vi "Write to Filter Log.vi"(8 "error in (no error)":errorcluster, 11 "Message Log in":refnum<class "Message Log.lvclass">) -> (0 "error out":errorcluster, 3 "Message Log out":refnum<class "Message Log.lvclass">)   [LabVIEW 2017, in "Message Log.lvclass"]
uses:
  Message Log.lvclass
  Message Log.lvclass/Message Log.ctl
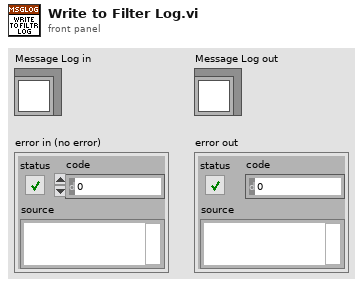
[diagram p1: front panel]
types:
  T1 = typedef "Message Log.lvclass/Message Log Filter Data.ctl" = cluster{"Element":string, "Column":T2, "Filter Type":T3}
  T2 = typedef "Message Log.lvclass/Message Log Columns.ctl" = enum16{"Count (sec)", "Time/Date", "Enque Worker", "Enque Case", "Deque Worker", "Deque Case", "Priority", "Message"}
  T3 = typedef "Message Log.lvclass/String Filter Type.ctl" = enum16{"string only", "match pattern"}
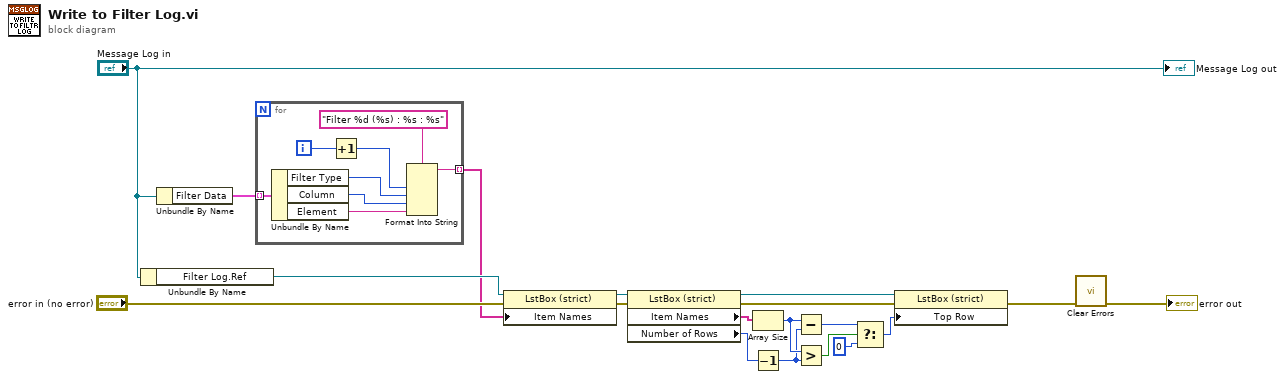
[diagram p0: block diagram]
diagram:
  n1 = Unbundle By Name("Message Log in") -> ("Filter Log.Ref"=w19:refnum<vi>)
  n2 = Unbundle By Name("Message Log in") -> ("Filter Data"=w5:T1[])
  n3 = for {
    tunnel: w5 -> [w24] mode=indexing
    tunnel: [w21] -> w2 mode=indexing
    i -> [w26]
    n4 = Unbundle By Name(w24) -> ("Filter Type"=w23:T3, "Column"=w20:T2, "Element"=w22:string)
    n5 = Increment(x=w26) -> (x+1=w25:i32)
    n6 = Format Into String(format string="Filter %d (%s) : %s : %s", w25, w23, w20, w22) -> (resulting string=w21:string)  [unwired: 2 in, 1 out]
  }
  n7 = property class="LstBox (strict)"(reference=w19, error in="error in (no error)", "Item Names"=w2) -> (reference out=w9:refnum<vi>, error out=w7:errorcluster)
  n8 = property class="LstBox (strict)"(reference=w9, error in=w7) -> (reference out=w8:refnum<vi>, error out=w6:errorcluster, "Item Names"=w14:string[], "Number of Rows"=w13:u32)
  n9 = Array Size(array=w14) -> (size(s)=w17:i32)
  n10 = Decrement(x=w13) -> (x-1=w11:u32)
  n11 = Subtract(x=w17, y=w11) -> (x-y=w16:u32)
  n12 = Greater?(x=w17, y=w11) -> (0:w18:bool)
  n13 = Select(t=w16, s=w18, f=u32 0) -> (s? t:f=w12:u32)
  n14 = property class="LstBox (strict)"(reference=w8, error in=w6, "Top Row"=w12) -> (error out=w10:errorcluster)  [unwired: 1 out]
  n15 = call <vilib>:"Clear Errors.vi"("error in (no error)"=w10) -> ("error out"=→"error out":errorcluster)  [unwired: 5 in, 1 out]
  "Message Log out" <- "Message Log in"
